vi "DrawScore.vi"(8 "error in (no error)":errorcluster, 9 "SnakeData":T1, 11 "Snake in":refnum<class "SnakeGame.lvclass">) -> (0 "error out":errorcluster, 3 "Snake out":refnum<class "SnakeGame.lvclass">)   [LabVIEW 2019, in "RT_Game.lvlib" / "SnakeGame.lvclass"]
uses:
  SnakeGame.lvclass
  C:/Users/FreshBob/Dropbox/VIs/myRIO_GameConsole/RT/RT_Game/Game/Game.lvclass
  SnakeData.ctl
  Direction.ctl
  Game/Coordinate.ctl
  CoordinateData.ctl
  Game/Game.lvclass
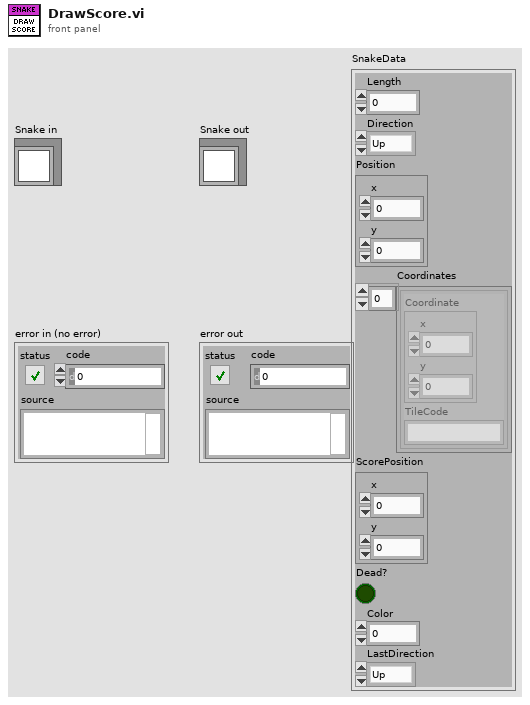
[diagram p1: front panel]
types:
  T1 = typedef "RT_Game.lvlib/SnakeGame.lvclass/SnakeData.ctl" = cluster{"Length":i16, "Direction":T2, "Position":T3, "Coordinates":T4[], "ScorePosition":T3, "Dead?":bool, "Color":fxp<+,3,3>, "LastDirection":T2}
  T2 = typedef "RT_Game.lvlib/SnakeGame.lvclass/Direction.ctl" = enum16{"Up", "Left", "Down", "Right"}
  T3 = typedef "RT_Game.lvlib/Game.lvclass/Coordinate.ctl" = cluster{"x":i16, "y":i16}
  T4 = typedef "RT_Game.lvlib/SnakeGame.lvclass/CoordinateData.ctl" = cluster{"Coordinate":T3, "TileCode":string}
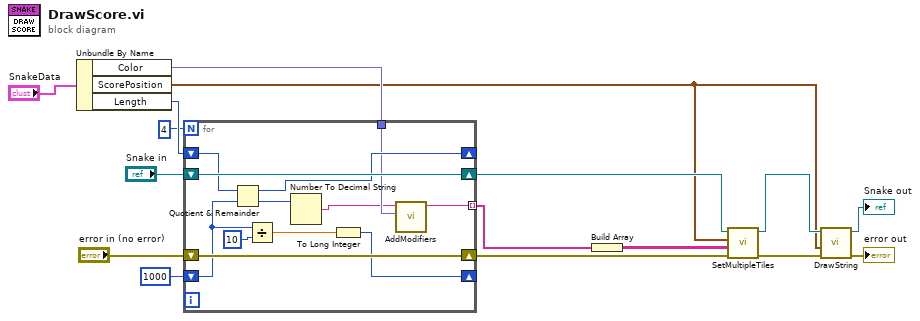
[diagram p0: block diagram]
diagram:
  n1 = Unbundle By Name("SnakeData") -> ("Color"=w4:fxp<+,3,3>, "ScorePosition"=w2:T3, "Length"=w16:i16)
  n2 = for {
    N: 4 -> [_]
    shift-right: [w28] -> w12
    shift-left: "error in (no error)" -> [w28]
    shift-right: [w27] -> w6
    shift-left: "Snake in" -> [w27]
    shift-right: [w20] -> _
    shift-left: 1000 -> [w26]
    shift-right: [w24] -> _
    shift-left: w16 -> [w23]
    tunnel: w4 -> [w18]
    tunnel: [w19] -> w3 mode=indexing
    n3 = Quotient & Remainder(x=w23, y=w26) -> (x-y*floor(x/y)=w24:i32, floor(x/y)=w25:i32)
    n4 = Divide(x=w26, y=10) -> (x/y=w21:dbl)
    n5 = Number To Decimal String(number=w25) -> (decimal integer string=w17:string)  [unwired: 1 in]
    n6 = To Long Integer(number=w21) -> (32bit integer=w20:i32)
    n7 = call "AddModifiers.vi"("ReplaceColor (1=red)"=w18, "String in"=w17) -> ("String out"=w19:string)  [unwired: 9 in]
  }
  n8 = Build Array(w3) -> (w1:string[][])
  n9 = call "SetMultipleTiles.vi"("error in (no error)"=w12, "TileCodes"=w1, "Position"=w2, "Game in"=w6) -> ("error out"=w7:errorcluster, "Game out"=w5:refnum<class "SnakeGame.lvclass">)  [unwired: 6 in]
  n10 = call "DrawString.vi"("error in (no error)"=w7, "Coordinate"=w2, "RT_Game.lvlib:Game.lvclass"=w5) -> ("error out"=→"error out":errorcluster, "RT_Game.lvlib:Game.lvclass 2"=→"Snake out":refnum<class "SnakeGame.lvclass">)  [unwired: 7 in]
